vi "PlungeMap_FBL.vi"(11 "Input (pA)":dbl) -> (3 "output":dbl)   [LabVIEW 2019]
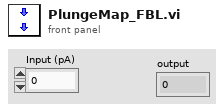
[diagram p1: front panel]
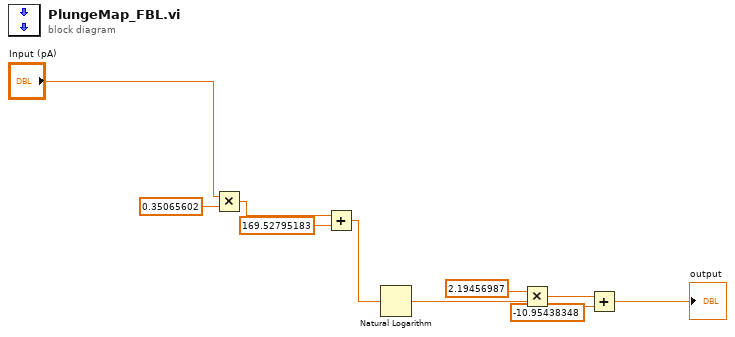
[diagram p0: block diagram]
diagram:
  n1 = Multiply(x="Input (pA)", y=0.35065602) -> (x*y=w8:dbl)
  n2 = Add(x=w8, y=169.52795183) -> (x+y=w6:dbl)
  n3 = Natural Logarithm(1:w6) -> (0:w5:dbl)
  n4 = Multiply(x=2.19456987, y=w5) -> (x*y=w3:dbl)
  n5 = Add(x=w3, y=-10.95438348) -> (x+y=→"output":dbl)
